vi "Render.vi"(8 "error in (no error)":errorcluster, 10 "String in":string, 11 "Footnote in":refnum<class "FootnoteReference.lvclass">) -> (0 "error out":errorcluster, 2 "String out":string, 3 "Footnote out":refnum<class "FootnoteReference.lvclass">)   [LabVIEW 2021, in "LvMarkdown.lvlib" / "FootnoteReference.lvclass"]
uses:
  FootnoteReference.lvclass
  FootnoteReference.lvclass/FootnoteReference.ctl
  GetReference.vi
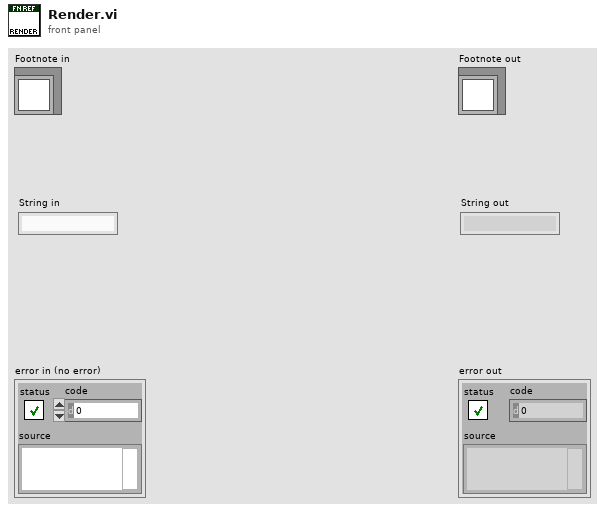
[diagram p1: front panel]
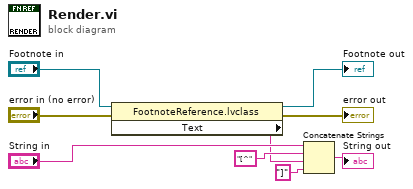
[diagram p0: block diagram]
diagram:
  n1 = property class="FootnoteReference.lvclass"(reference="Footnote in", error in="error in (no error)") -> (reference out=→"Footnote out":refnum<class "FootnoteReference.lvclass">, error out=→"error out":errorcluster, "Text"=w5:string)
  n2 = Concatenate Strings("String in", "[^" ("string"), w5, "]" ("string")) -> (→"String out":string)
